vi "Defer Panel Updates.vi"(7 "Action":enum16{"Init", "Freeze", "Unfreeze"}(ring)=enum."Unfreeze", 8 "Error In":errorcluster, 11 "reference":refnum<vi>) -> (0 "Error Out":errorcluster)   [LabVIEW 2017]
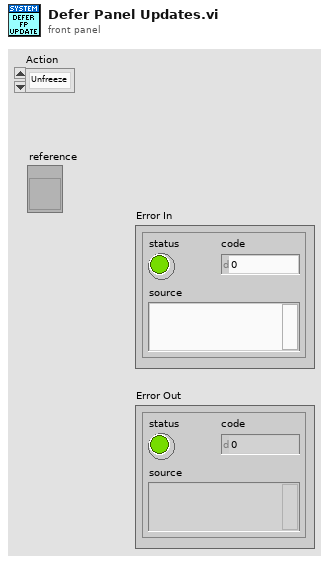
[diagram p1: front panel]
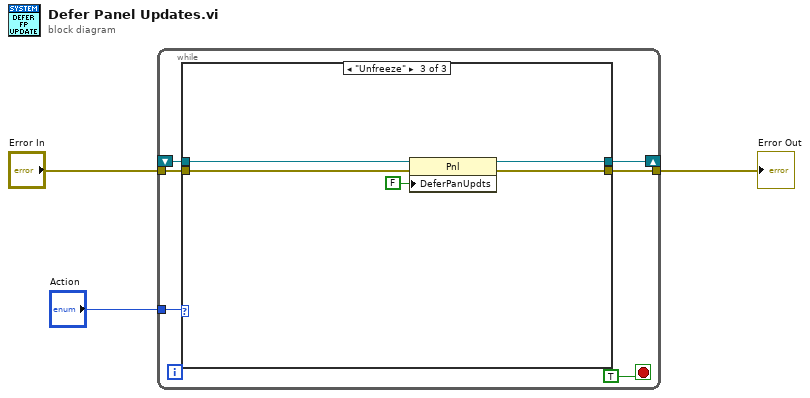
[diagram p0: block diagram]
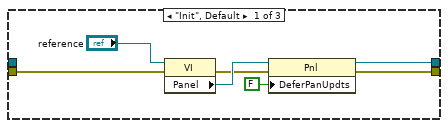
[diagram p2: hidden frame]
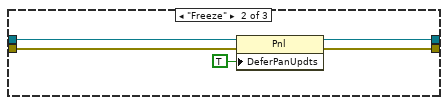
[diagram p3: hidden frame]
diagram:
  n1 = while {
    tunnel: "Action" -> [w8]
    shift-right: [w7] -> _
    shift-left: _ -> [w6]
    tunnel: "Error In" -> [w5]
    tunnel: [w4] -> w1
    stop <- TRUE stop-if-true
    n2 = case shown="\"Unfreeze\"" w8 {
      tunnel: [w14 w20 w25] -> w7
      tunnel: w6 -> [_ w21 w26]
      tunnel: w5 -> [w11 w19 w24]
      tunnel: [w10 w18 w23] -> w4
      frame "Init", Default {
        n3 = property class="VI"(reference="reference", error in=w11) -> (error out=w12:errorcluster, "Panel"=w15:refnum<vi>)  [unwired: 1 out]
        n4 = property class="Pnl"(reference=w15, error in=w12, "DeferPanUpdts"=FALSE ("Defer Panel Updates")) -> (reference out=w14:refnum<vi>, error out=w10:errorcluster)
      }
      frame "Freeze" {
        n5 = property class="Pnl"(reference=w21, error in=w19, "DeferPanUpdts"=TRUE ("Defer Panel Updates")) -> (reference out=w20:refnum<vi>, error out=w18:errorcluster)
      }
      frame "Unfreeze" {
        n6 = property class="Pnl"(reference=w26, error in=w24, "DeferPanUpdts"=FALSE ("Defer Panel Updates")) -> (reference out=w25:refnum<vi>, error out=w23:errorcluster)
      }
    }
  }
  "Error Out" <- w1
